vi "Simulation-04.vi"() -> ()   [LabVIEW 2020]
uses:
  librarian_class/typedefs/book_state--enum.ctl
  shared/request--enum.ctl
  librarian_class/librarian.lvclass
  client_class/client.lvclass
panel:
  out "success":bool
  out "lib error out":errorcluster
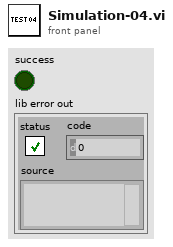
[diagram p1: front panel]
types:
  T1 = typedef "request--enum.ctl" = enum16{"CHECKIN", "CHECKOUT"}
  T2 = typedef "librarian.lvclass/book_state--enum.ctl" = enum16{"CHECKEDIN", "CHECKEDOUT", "DAMAGED"}
  T3 = typedef "message--cluster.ctl" = cluster{"header":string, "cmd":T1, "title":string, "book":string}
  T4 = typedef "librarian.lvclass/lib_map_value--cluster.ctl" = cluster{"book state":T2, "text":string, "hash":string}
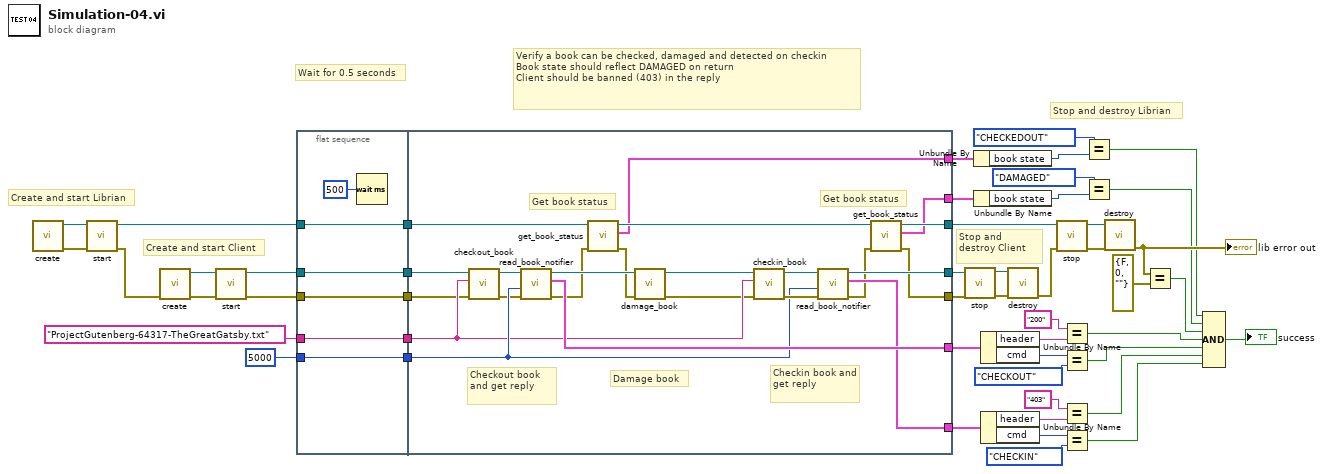
[diagram p0: block diagram]
diagram:
  # "Verify a book can be checked, damaged and detected on checkin\nBook state should reflect DAMAGED on return\nClient should be banned (403) in the reply"
  # "Stop and destroy Client"
  # "Stop and destroy Librian"
  # "Wait for 0.5 seconds"
  # "Create and start Client"
  # "Create and start Librian"
  n1 = call "create.vi"() -> ("error out"=w48:errorcluster, "librarian_sm out"=w49:refnum<class "librarian.lvclass">)  [unwired: 10 in]
  n2 = call "start.vi"("error in (no error)"=w48, "librarian_sm in"=w49) -> ("error out"=w28:errorcluster, "librarian_sm out"=w39:refnum<class "librarian.lvclass">)  [unwired: 8 in]
  n3 = call "create.vi"("error in (no error)"=w28) -> ("error out"=w44:errorcluster, "librarian_sm out"=w45:refnum<class "client.lvclass">)  [unwired: 9 in]
  n4 = call "start.vi"("error in (no error)"=w44, "librarian_sm in"=w45) -> ("error out"=w41:errorcluster, "librarian_sm out"=w40:refnum<class "client.lvclass">)  [unwired: 8 in]
  n5 = flat-sequence {
    tunnel: "ProjectGutenberg-64317-TheGreatGatsby.txt" ("book title") -> [w50]
    tunnel: 5000 ("timeout in ms (-1)") -> [w53]
    tunnel: w39 -> [w54]
    tunnel: w40 -> [w55]
    tunnel: w41 -> [w51]
    tunnel: [w51] -> w33
    tunnel: [w55] -> w32
    tunnel: [w54] -> w31
    tunnel: [w53] -> w30
    tunnel: [w50] -> w29
    tunnel: [w78] -> w12
    tunnel: [w58] -> w36
    tunnel: [w73] -> w37
    tunnel: [w62] -> w38
    tunnel: [w72] -> w11
    tunnel: w29 -> [w74]
    tunnel: w30 -> [w75]
    tunnel: w31 -> [w64]
    tunnel: w32 -> [w70]
    tunnel: w33 -> [w71]
    tunnel: [w57] -> w21
    tunnel: [w56] -> w22
    frame #0 {
      n6 = Wait (ms)(milliseconds to wait=u32 500) -> ()  [unwired: 1 out]
    }
    frame #1 {
      # "Damage book"
      # "Checkin book and get reply"
      # "Get book status"
      # "Get book status"
      # "Checkout book and get reply"
      n7 = call "checkout_book.vi"("error in (no error)"=w71, "book title"=w74, "client in"=w70) -> ("error out"=w68:errorcluster, "client out"=w69:refnum<class "client.lvclass">)  [unwired: 7 in]
      n8 = call "read_book_notifier.vi"("error in (no error)"=w68, "timeout in ms (-1)"=w75, "client in"=w69) -> ("error out"=w61:errorcluster, "msg"=w78:T3, "client out"=w67:refnum<class "client.lvclass">)  [unwired: 6 in]
      n9 = call "get_book_status.vi"("error in (no error)"=w61, "librarian in"=w64) -> ("error out"=w60:errorcluster, "book status"=w56:T4, "librarian out"=w63:refnum<class "librarian.lvclass">)  [unwired: 7 in]
      n10 = call "damage_book.vi"("error in (no error)"=w60, "client in"=w67) -> ("error out"=w65:errorcluster, "client out"=w66:refnum<class "client.lvclass">)  [unwired: 8 in]
      n11 = call "checkin_book.vi"("error in (no error)"=w65, "book title"=w74, "client in"=w66) -> ("error out"=w76:errorcluster, "client out"=w77:refnum<class "client.lvclass">)  [unwired: 7 in]
      n12 = call "read_book_notifier.vi"("error in (no error)"=w76, "timeout in ms (-1)"=w75, "client in"=w77) -> ("error out"=w59:errorcluster, "msg"=w72:T3, "client out"=w73:refnum<class "client.lvclass">)  [unwired: 6 in]
      n13 = call "get_book_status.vi"("error in (no error)"=w59, "librarian in"=w63) -> ("error out"=w58:errorcluster, "book status"=w57:T4, "librarian out"=w62:refnum<class "librarian.lvclass">)  [unwired: 7 in]
    }
  }
  n14 = call "stop.vi"("error in (no error)"=w36, "librarian_sm in"=w37) -> ("error out"=w42:errorcluster, "librarian_sm out"=w43:refnum<class "client.lvclass">)  [unwired: 8 in]
  n15 = Unbundle By Name(w22) -> ("book state"=w26:T2)
  n16 = Unbundle By Name(w21) -> ("book state"=w23:T2)
  n17 = Unbundle By Name(w12) -> ("header"=w20:string, "cmd"=w18:T1)
  n18 = Unbundle By Name(w11) -> ("header"=w13:string, "cmd"=w15:T1)
  n19 = call "destroy.vi"("error in (no error)"=w42, "librarian_sm in"=w43) -> ("error out"=w27:errorcluster)  [unwired: 8 in, 1 out]
  n20 = call "stop.vi"("error in (no error)"=w27, "librarian_sm in"=w38) -> ("error out"=w46:errorcluster, "librarian_sm out"=w47:refnum<class "librarian.lvclass">)  [unwired: 8 in]
  n21 = Equal?(x="200", y=w20) -> (x = y?=w5:bool)
  n22 = Equal?(x=w18, y=request--enum."CHECKOUT") -> (x = y?=w4:bool)
  n23 = Equal?(x="403", y=w13) -> (x = y?=w3:bool)
  n24 = Equal?(x=w15, y=request--enum."CHECKIN") -> (x = y?=w2:bool)
  n25 = Equal?(x=book_state--enum."CHECKEDOUT", y=w26) -> (x = y?=w8:bool)
  n26 = Equal?(x=book_state--enum."DAMAGED", y=w23) -> (x = y?=w7:bool)
  n27 = call "destroy.vi"("error in (no error)"=w46, "librarian_sm in"=w47) -> ("error out"=w9:errorcluster)  [unwired: 8 in, 1 out]
  "lib error out" <- w9
  n28 = Equal?(x=w9, y=errorcluster {"status"=FALSE, "code"=0, "source"=""}) -> (x = y?=w6:bool)
  n29 = Compound Arithmetic op=AND(w8, w7, w6, w5, w4, w3, w2) -> (→"success":bool)
